vi "创建数据表.vi"(8 "error in (no error)":errorcluster) -> (0 "error out":errorcluster)   [LabVIEW 2016, in "数据查询.lvlib"]
uses:
  <vilib>/addons/database/Auxilliary.llb/DB Tools Column Info.ctl
  <vilib>/addons/database/Auxilliary.llb/DB Tools DataTypes.ctl
  <vilib>/addons/database/Connection.llb/DB Tools Open Connec (String).vi
  <userlib>/_LVST/sqlite_api/Core/Tables/SQLite_Drop Table.vi
  <userlib>/_LVST/sqlite_api/Core/Tables/SQLite_Create Table.vi
  <vilib>/addons/database/NI_Database_API.lvlib
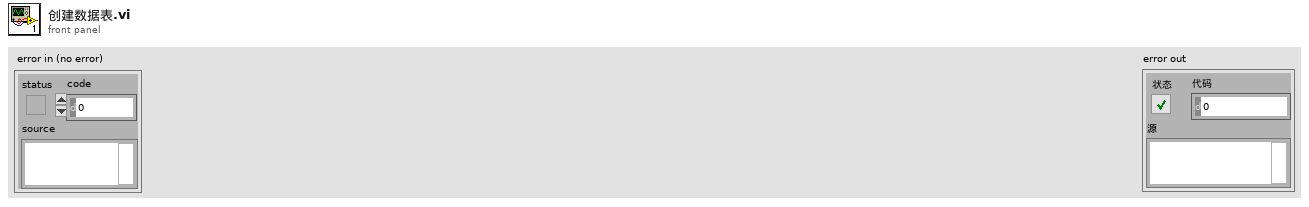
[diagram p1: front panel]
types:
  T1 = typedef "NI_Database_API.lvlib/DB Tools Column Info.ctl" = cluster{"column name":string, "data type":T2, "size":i32, "allow null?":bool}
  T2 = typedef "NI_Database_API.lvlib/DB Tools DataTypes.ctl" = enum16{"String", "Long (I32)", "Single (SGL)", "Double (DBL)", "Date/Time", "Binary"}
  T3 = typedef "数据库类型.ctl" = enum16{"Access", "SQLite"}
  T4 = typedef "NI_Database_API.lvlib/Conn ObjectReference.ctl" = refnum<k1>
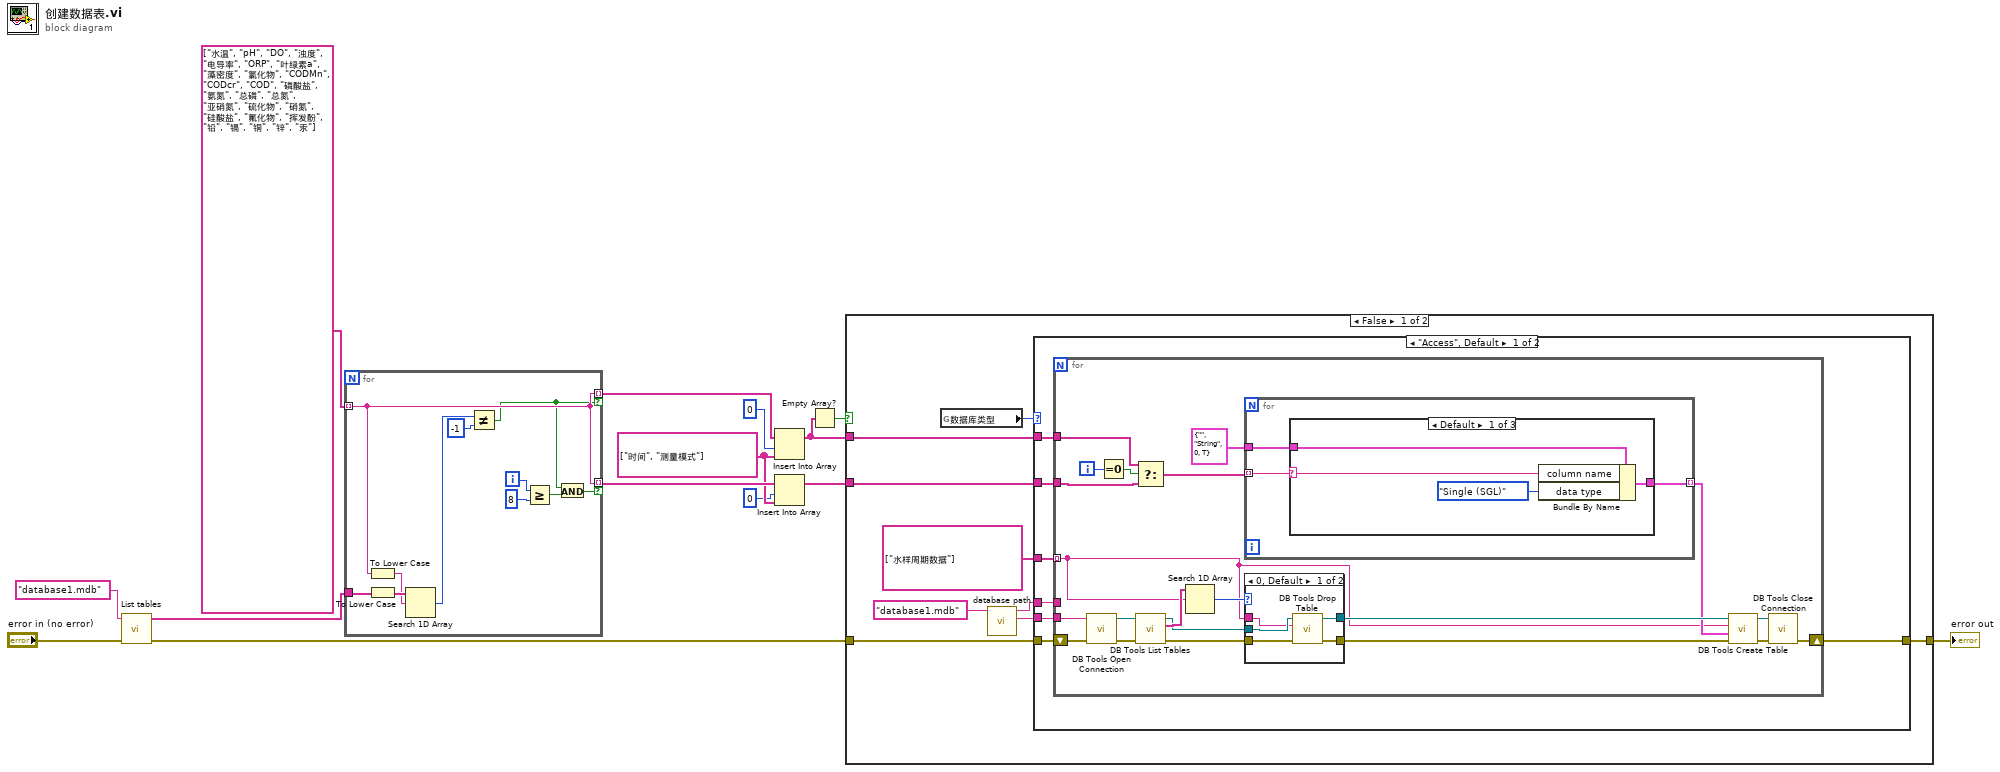
[diagram p0: block diagram]
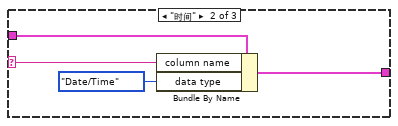
[diagram p2: hidden frame]
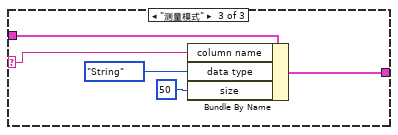
[diagram p3: hidden frame]
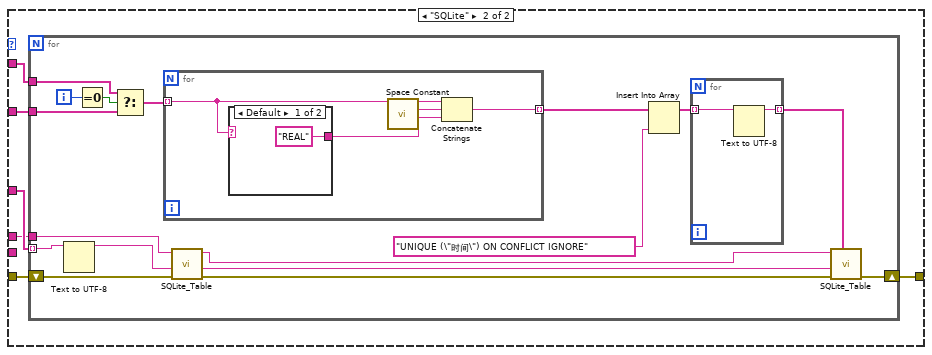
[diagram p5: hidden frame]
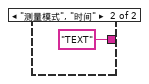
[diagram p6: hidden frame]
diagram:
  w9 = string[] ["时间", "测量模式"]
  n1 = call "List tables.vi"("error in (no error)"="error in (no error)", "database"="database1.mdb") -> ("error out"=w6:errorcluster, "tables"=w14:string[])  [unwired: 8 in]
  n2 = for {
    tunnel: string[] ["水温", "pH", "DO", "浊度", "电导率", "ORP", "叶绿素a", "藻密度", "氯化物", "CODMn", "CODcr", "COD", "磷酸盐", "氨氮", "总磷", "总氮", "亚硝氮", "硫化物", "硝氮", "硅酸盐", "氟化物", "挥发酚", "铅", "镉", "铜", "锌", "汞"] -> [w22] mode=indexing
    tunnel: w14 -> [w25]
    tunnel: [w22] -> w13 mode=indexing if=w17
    tunnel: [w22] -> w10 mode=indexing if=w18
    i -> [w21]
    n3 = To Lower Case(string=w22) -> (all lower case string=w15:string)
    n4 = To Lower Case(string=w25) -> (all lower case string=w16:string[])
    n5 = Search 1D Array(1D array=w16, element=w15) -> (index of element=w24:i32)  [unwired: 1 in]
    n6 = Not Equal?(x=w24, y=-1 ("x")) -> (x != y?=w17:bool)
    n7 = Greater Or Equal?(x=w21, y=8) -> (x >= y?=w19:bool)
    n8 = And(x=w17, y=w19) -> (x .and. y?=w18:bool)
  }
  n9 = Insert Into Array(array=w13, index=0 ("索引"), new element=w9) -> (w2:string[])
  n10 = Insert Into Array(array=w10, index=0 ("索引"), new element=w9) -> (w5:string[])
  n11 = Empty Array?(array=w2) -> (empty?=w1:bool)
  n12 = case shown="False" w1 {
    tunnel: w6 -> [w34 w117]
    tunnel: w5 -> [w32 _]
    tunnel: [w31 w117] -> w3
    tunnel: w2 -> [w26 _]
    frame False {
      n13 = global read "外部调用接口全局变量.vi" "数据库类型"() -> (w27:T3)
      n14 = call "database path.vi"("database"="database1.mdb") -> ("Connection information"=w28:string, "Path out"=w29:string)  [unwired: 9 in]
      n15 = case shown="\"Access\", Default" w27 {
        tunnel: w26 -> [w41 w90]
        tunnel: w34 -> [w40 w87]
        tunnel: [w39 w88] -> w31
        tunnel: string[] ["水样周期数据"] -> [w38 w91]
        tunnel: w32 -> [w37 w89]
        tunnel: w29 -> [w36 w86]
        tunnel: w28 -> [w35 _]
        frame "Access", Default {
          n16 = for {
            tunnel: w41 -> [w45]
            shift-right: [w49] -> w39
            shift-left: w40 -> [w50]
            tunnel: w38 -> [w48] mode=indexing
            tunnel: w37 -> [w44]
            tunnel: w36 -> [_]
            tunnel: w35 -> [w42]
            i -> [w47]
            n17 = call-poly <vilib>:"DB Tools Open Connection.vi"("error in (no error)"=w50, "connection information"=w42) -> ("error out"=w62:errorcluster, "connection reference"=w61:T4)  [unwired: 6 in]
            n18 = Equal To 0?(x=w47) -> (x = 0?=w46:bool)
            n19 = Select(t=w45, s=w46, f=w44) -> (s? t:f=w43:string[])
            n20 = call <vilib>:"DB Tools List Tables.vi"("error in (no error)"=w62, "connection reference"=w61) -> ("error out"=w56:errorcluster, "tables"=w60:string[], "connection reference out"=w58:T4)  [unwired: 3 in]
            n21 = Search 1D Array(1D array=w60, element=w48) -> (index of element=w59:i32)  [unwired: 1 in]
            n22 = for {
              tunnel: w43 -> [w65] mode=indexing
              tunnel: T1 {"column name"="", "data type"=enum."String", "size"=0, "allow null?"=TRUE} ("column information") -> [w64]
              tunnel: [w63] -> w51 mode=indexing
              n23 = case shown="Default" w65 {
                selector: w65 -> [w68 w72 w77]
                tunnel: w64 -> [w69 w73 w78]
                tunnel: [w67 w71 w76] -> w63
                frame Default {
                  n24 = Bundle By Name(cluster=w69, "column name"=w68, "data type"=DB_Tools_DataTypes."Single (SGL)") -> (w67:T1)
                }
                frame "时间" {
                  n25 = Bundle By Name(cluster=w73, "column name"=w72, "data type"=DB_Tools_DataTypes."Date/Time") -> (w71:T1)
                }
                frame "测量模式" {
                  n26 = Bundle By Name(cluster=w78, "column name"=w77, "data type"=DB_Tools_DataTypes."String", "size"=50) -> (w76:T1)
                }
              }
            }
            n27 = case shown="0, Default" w59 {
              tunnel: w58 -> [w83 w85]
              tunnel: [w82 w85] -> w57
              tunnel: w56 -> [w81 w84]
              tunnel: [w80 w84] -> w55
              tunnel: w48 -> [w79 _]
              frame 0, Default {
                n28 = call <vilib>:"DB Tools Drop Table.vi"("error in (no error)"=w81, "table"=w79, "connection reference"=w83) -> ("error out"=w80:errorcluster, "connection reference out"=w82:T4)  [unwired: 5 in]
              }
              frame -1 {
              }
            }
            n29 = call <vilib>:"DB Tools Create Table.vi"("error in (no error)"=w55, "column information"=w51, "table"=w48, "connection reference"=w57) -> ("error out"=w53:errorcluster, "connection reference out"=w54:T4)  [unwired: 4 in]
            n30 = call <vilib>:"DB Tools Close Connection.vi"("error in (no error)"=w53, "connection reference"=w54) -> ("error out"=w49:errorcluster)  [unwired: 5 in]
          }
        }
        frame "SQLite" {
          n31 = for {
            tunnel: w86 -> [w96]
            tunnel: w91 -> [w95] mode=indexing
            tunnel: w90 -> [w103]
            tunnel: w89 -> [w102]
            shift-right: [w100] -> w88
            shift-left: w87 -> [w99]
            i -> [w105]
            n32 = Text to UTF-8(11:w95) -> (3:w94:string)  [unwired: 2 in, 1 out]
            n33 = Equal To 0?(x=w105) -> (x = 0?=w104:bool)
            n34 = Select(t=w103, s=w104, f=w102) -> (s? t:f=w101:string[])
            n35 = for {
              tunnel: w101 -> [w114] mode=indexing
              tunnel: [w111] -> w97 mode=indexing
              n36 = case shown="Default" w114 {
                tunnel: ["REAL" "TEXT"] -> w112
                frame Default {
                }
                frame "测量模式", "时间" {
                }
              }
              n37 = call <vilib>:"Space Constant.vi"() -> ("String"=w113:string)
              n38 = Concatenate Strings(w114, w113, w112) -> (w111:string)
            }
            n39 = call-poly <userlib>:"SQLite_Table.vi"("DB Path"=w96, "Table Name"=w94, "error in (no error)"=w99) -> ("DB Path Out"=w108:string, "Table Name Out"=w106:string, "error out"=w107:errorcluster)  [unwired: 5 in]
            n40 = Insert Into Array(array=w97, new element="UNIQUE (\"时间\") ON CONFLICT IGNORE" ("新元素/子数组")) -> (w93:string[])  [unwired: 1 in]
            n41 = for {
              tunnel: w93 -> [w110] mode=indexing
              tunnel: [w109] -> w92 mode=indexing
              n42 = Text to UTF-8(11:w110) -> (3:w109:string)  [unwired: 2 in, 1 out]
            }
            n43 = call-poly <userlib>:"SQLite_Table.vi"("DB Path"=w108, "Table Name"=w106, "error in (no error)"=w107, "Columns"=w92) -> ("error out"=w100:errorcluster)  [unwired: 4 in, 2 out]
          }
        }
      }
    }
    frame True {
    }
  }
  "error out" <- w3
